vi "State(FGV).vi"(8 "Error In":errorcluster, 9 "Action":enum16{"Set", "Get"}(ring), 11 "input state":T2) -> (0 "Error Out":errorcluster, 2 "Output \nIndicator":T1 caption="Z     Y     X", 3 "output state":T2)   [LabVIEW 2023]
doc: "This VI realizes a functional global variable that stores the current state of the FSM."
uses:
  controls/Boolean output indicator.ctl
  controls/enum defining states.ctl
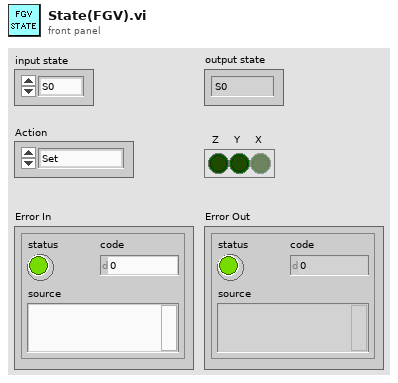
[diagram p1: front panel]
types:
  T1 = typedef "Boolean output indicator.ctl" = bool[]
  T2 = typedef "enum defining states.ctl" = enum16{"S0", "S1", "S2", "S3"}
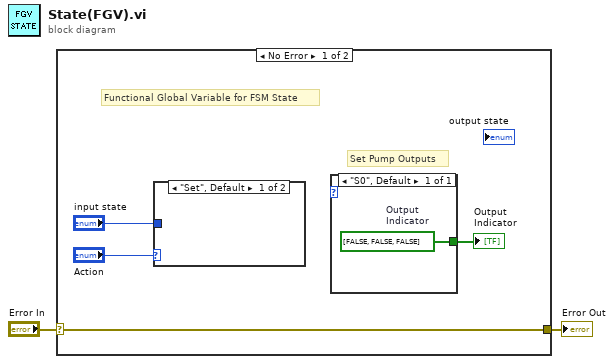
[diagram p0: block diagram]
diagram:
  n1 = case shown="No Error" "Error In" {
    selector: "Error In" -> [w5 w8]
    tunnel: [w5 w8] -> w1
    frame No Error {
      # "Set Pump Outputs"
      # "Functional Global Variable for FSM State"
      n2 = case shown="\"Set\", Default" "Action" {
        tunnel: "input state" -> [_ _]
        frame "Set", Default {
        }
        frame "Get" {
        }
      }
      n3 = case shown="\"S0\", Default" {
        selector: _ -> [_]
        tunnel: [w7] -> w3
        frame "S0", Default {
          w7 = T1 [FALSE, FALSE, FALSE]  # Output  Indicator
        }
      }
      "Output \nIndicator" <- w3
    }
    frame Error {
    }
  }
  "Error Out" <- w1
